vi "WPI_IMU_ADIS16448_Close.vi"(8 "error in":errorcluster, 11 "ADI IMU Interrupt DevRef":T1={"ADI IMU DevRef"={"DevStatus"={"status"=FALSE, "code"=0, "source"=""}, "Handle"=0, "SPI Bus"=enum."SPI On-Board, CS0", "Device Found"=FALSE, "Device Ready"=FALSE, "Yaw Axis"=enum."Z", "AHRS Algorithm"=enum."Complementary", "Serial"=0, "Lot ID 2"=0, "Lot ID 1"=0, "Product ID"=0}, "InterruptRef"={"DevStatus"={"status"=FALSE, "code"=0, "source"=""}, "InterruptIndex"=enum."0"}}) -> (0 "error out":errorcluster)   [LabVIEW 2016, in "FRC_ADIS16448_IMU.lvlib"]
doc: "Closes the ADIIMUDevRef and properly shuts down SPI communication between the RoboRIO and the ADI IMU MXP board."
uses:
  FRC_ADIS16448_IMU.lvlib
  WPI_IMU_ADIS16448_InterruptDevRef.ctl
  WPI_IMU_ADIS16448_IMUDevRef.ctl
  <vilib>/Rock Robotics/SystemInterfaces/spilib/spi_bus.ctl
  <vilib>/Rock Robotics/WPI/Interrupt/WPI_InterruptRef.ctl
  <vilib>/Rock Robotics/SystemInterfaces/Interrupt/FPGA_InterruptIndex.ctl
  <vilib>/Rock Robotics/WPI/SPI/WPI_SPIDevRef.ctl
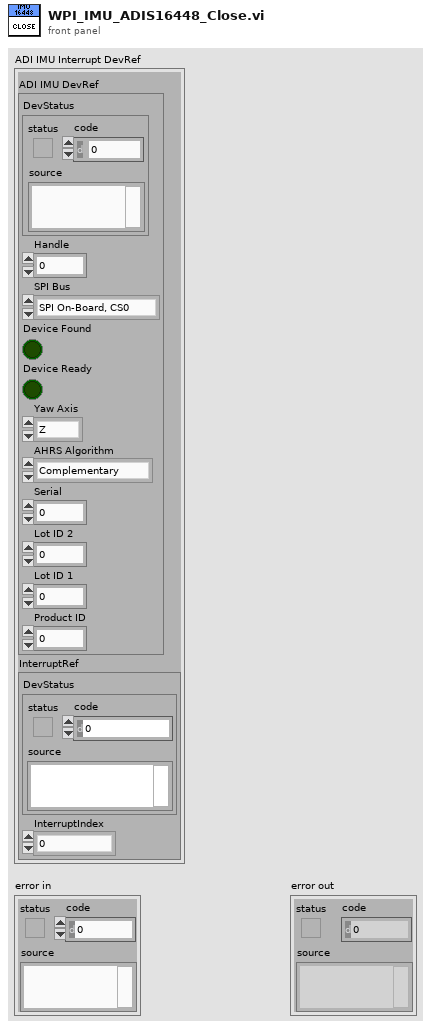
[diagram p1: front panel]
types:
  T1 = typedef "FRC_ADIS16448_IMU.lvlib/WPI_IMU_ADIS16448_InterruptDevRef.ctl" = cluster{"ADI IMU DevRef":T2, "InterruptRef":T4}
  T2 = typedef "FRC_ADIS16448_IMU.lvlib/WPI_IMU_ADIS16448_IMUDevRef.ctl" = cluster{"DevStatus":errorcluster, "Handle":i32, "SPI Bus":T3, "Device Found":bool, "Device Ready":bool, "Yaw Axis":enum16{"X", "Y", "Z"}, "AHRS Algorithm":enum16{"Complementary", "Madgwick"}, "Serial":u16, "Lot ID 2":u16, "Lot ID 1":u16, "Product ID":u16}
  T3 = typedef "spi_bus.ctl" = enum16{"SPI On-Board, CS0", "SPI On-Board, CS1", "SPI On-Board, CS2", "SPI On-Board, CS3", "SPI MXP", "Invalid"}
  T4 = typedef "WPI_InterruptRef.ctl" = cluster{"DevStatus":errorcluster, "InterruptIndex":T5}
  T5 = typedef "FPGA_InterruptIndex.ctl" = enum8{"0", "1", "2", "3", "4", "5", "6", "7", "Invalid"}
  T6 = typedef "WPI_SPIDevRef.ctl" = cluster{"DevStatus":errorcluster, "Handle":i32, "SPI Bus":T3}
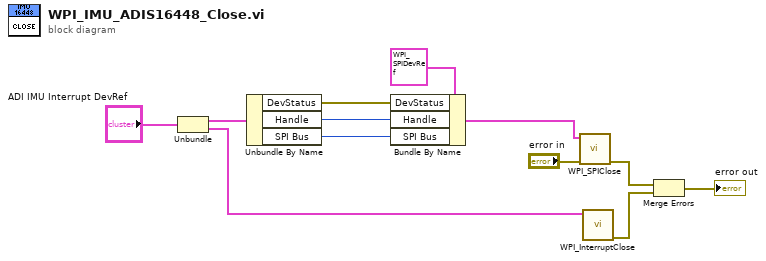
[diagram p0: block diagram]
diagram:
  n1 = Unbundle("ADI IMU Interrupt DevRef") -> ("ADI IMU DevRef"=w5:T2, "InterruptRef"=w4:T4)
  n2 = Unbundle By Name(w5) -> ("DevStatus"=w10:errorcluster, "Handle"=w9:i32, "SPI Bus"=w8:T3)
  n3 = Bundle By Name(cluster=T6 {"DevStatus"={"status"=FALSE, "code"=0, "source"=""}, "Handle"=0, "SPI Bus"=enum."SPI On-Board, CS0"} ("SPIDevRef"), "DevStatus"=w10, "Handle"=w9, "SPI Bus"=w8) -> (w7:T6)
  n4 = call <vilib>:"WPI_SPIClose.vi"("error in (no error)"="error in", "SPIDevRef"=w7) -> ("error out"=w3:errorcluster)  [unwired: 9 in]
  n5 = call <vilib>:"WPI_InterruptClose.vi"("InterruptRef"=w4) -> ("error out"=w2:errorcluster)  [unwired: 10 in]
  n6 = Merge Errors(w3, w2) -> (→"error out":errorcluster)
